vi "Picolog Thermocouple Basic.vi"() -> ()   [LabVIEW 2017]
uses:
  Controls/Thermocouple.ctl
  Controls/Temperature Units.ctl
  Controls/Fill Missing.ctl
  Controls/State Control.ctl
panel:
  in  "Tab Control":enum32{"Configuration", "Results"}(tab)=enum."Results"
  in  "Thermocouples":T1[](array[typedef])=[107, 32, 32, 32, 32, 32, 32, 32, 32, 32] items=["B"=98, "E"=101, "J"=106, "K"=107, "N"=110, "R"=114, "S"=115, "T"=116, "Voltage"=120, "Internal"=0, "Off"=32]
  in  "Mains Frequency":i16(ring) items=["50 Hz", "60 Hz"]
  in  "Unit":T2
  in  "Sampling Interval [s]":dbl=0.20000000000000004 min=0.1 max=100.0 step=0.1 format="%#_13g"
  in  "Fill Missing Points":T3 items=["QNaN", "Previous"]
  in  "Buffer Length":i32=128
  in  "Update Rate [s]":dbl=0.20000000000000004 min=0.1 max=10.0 step=0.1
  out "Actual Interval [s]":dbl=0.20000000000000004
  out "Error":errorcluster
  out "Temperature":waveform(dbl)[](graph)=[{"t0"=timestamp(3630055576.922543 s since 1904-01-01), "dt"=0.20000000000000284, "Y"=[23.393163681030273], "attributes"=variant("NI_ChannelName"=variant(string "Cold Junction"))}, {"t0"=timestamp(3630055576.922543 s since 1904-01-01), "dt"=0.20000000000000284, "Y"=[23.27175521850586], "attributes"=variant("NI_ChannelName"=variant(string "Channel 1"))}]
  in  "Stop":bool
  # "Temperature Measurement - PicoLog Thermocouple"
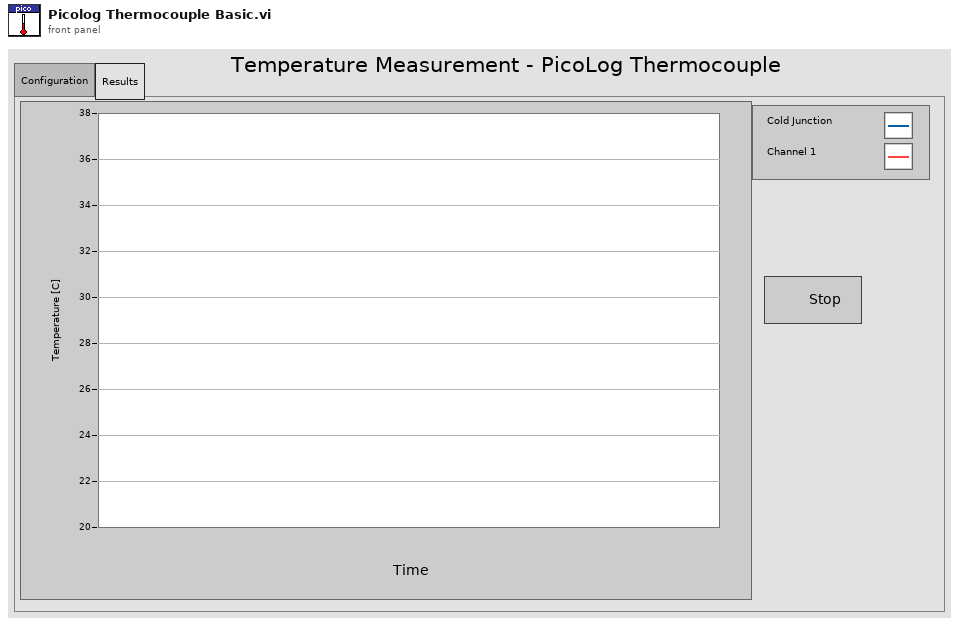
[diagram p1: front panel]
types:
  T1 = typedef "Thermocouple.ctl" = i8
  T2 = typedef "Temperature Units.ctl" = enum16{"°C", "°F", "K", "°R"}
  T3 = typedef "Fill Missing.ctl" = i16
  T4 = typedef "State Control.ctl" = enum16{"Initialize", "Idle", "Acquire", "Display", "Shutdown", "Quit", "Error"}
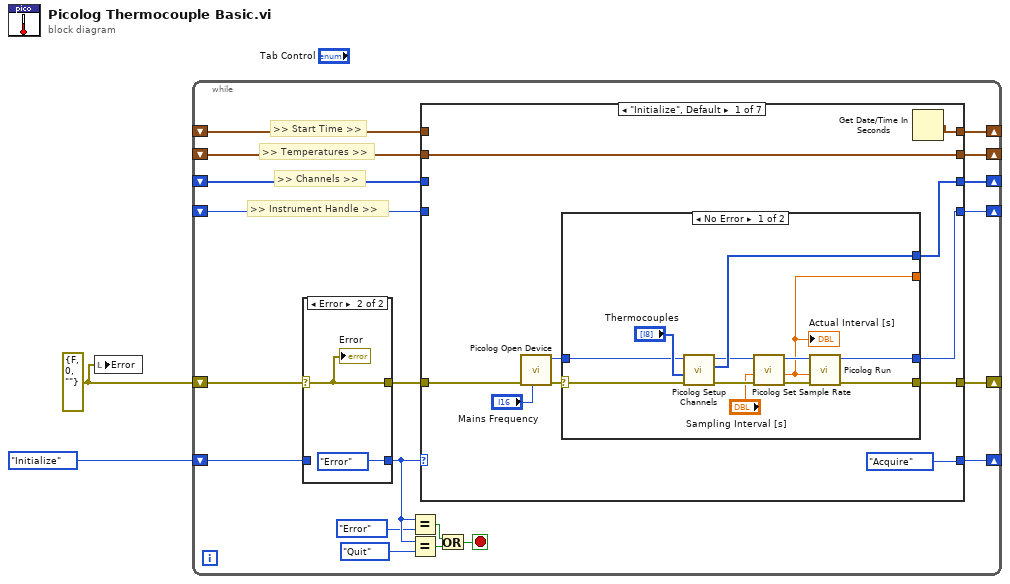
[diagram p0: block diagram]
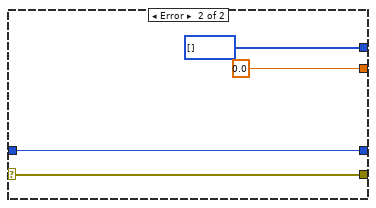
[diagram p3: hidden frame]
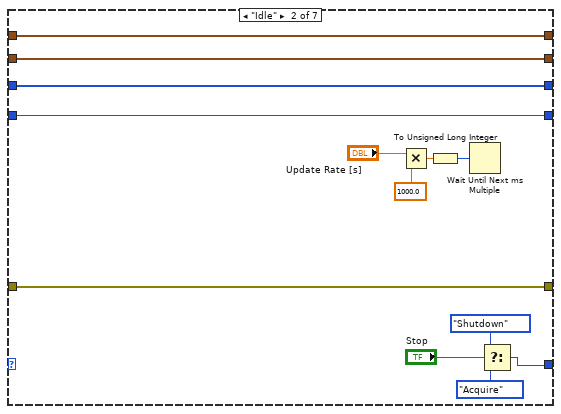
[diagram p4: hidden frame]
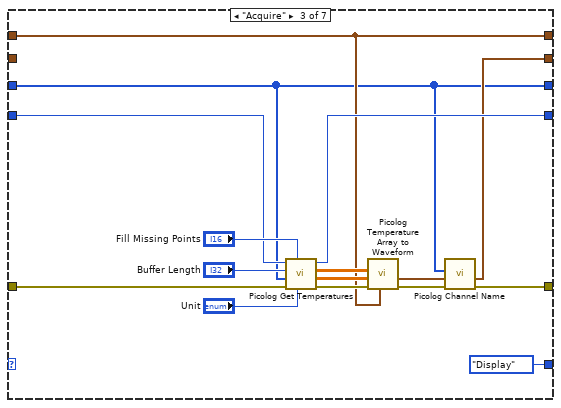
[diagram p5: hidden frame]
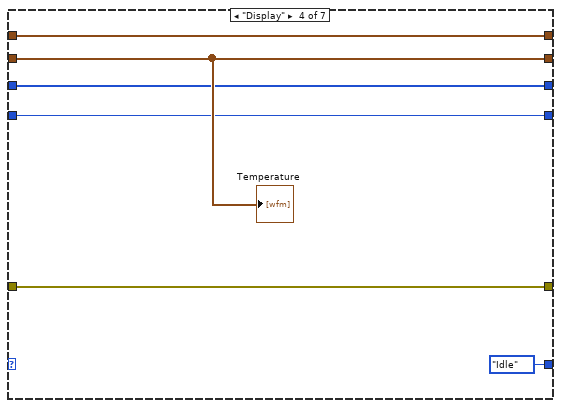
[diagram p6: hidden frame]
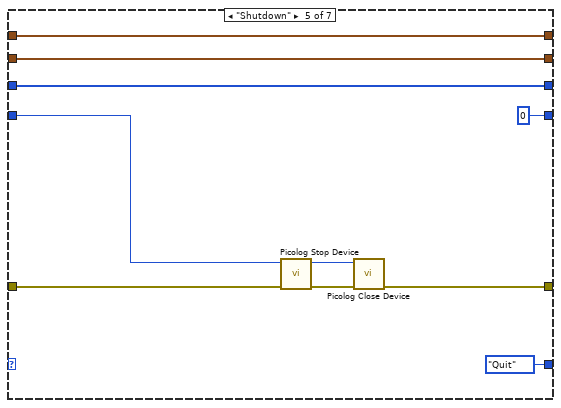
[diagram p7: hidden frame]
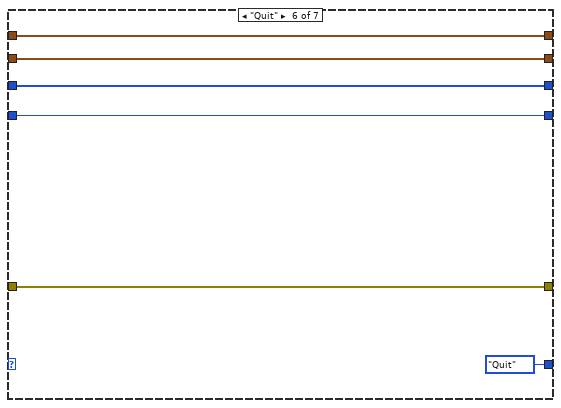
[diagram p8: hidden frame]
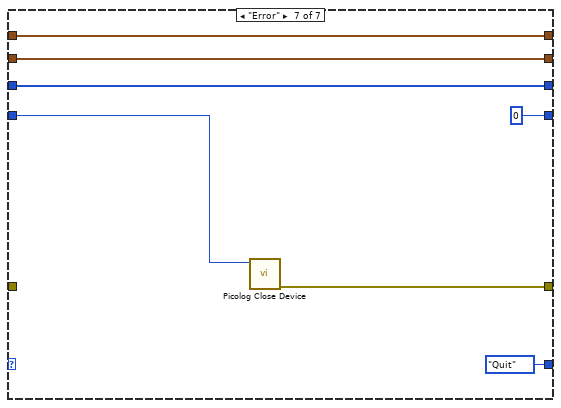
[diagram p9: hidden frame]
diagram:
  w1 = errorcluster {"status"=FALSE, "code"=0, "source"=""} ("Error Out")
  n1 = local write "Error"(w1) -> ()
  n2 = while {
    shift-right: [w12] -> _
    shift-left: _ -> [w20]
    shift-right: [w21] -> _
    shift-left: w1 -> [w5]
    shift-right: [w19] -> _
    shift-left: State_Control."Initialize" ("State") -> [w13]
    shift-right: [w18] -> _
    shift-left: _ -> [w17]
    shift-right: [w16] -> _
    shift-left: _ -> [w15]
    shift-right: [w4] -> _
    shift-left: _ -> [w3]
    stop <- w6 stop-if-true
    # ">> Start Time >>"
    # ">> Temperatures >>"
    # ">> Instrument Handle >>"
    # ">> Channels >>"
    n3 = case shown="Error" w5 {
      selector: w5 -> [w23 w24]
      tunnel: [w23 w24] -> w14
      tunnel: w13 -> [w22 _]
      tunnel: [w22 State_Control."Error" ("State")] -> w10
      frame No Error {
      }
      frame Error {
        "Error" <- w24
      }
    }
    n4 = Equal?(x=w10, y=State_Control."Error") -> (x = y?=w8:bool)
    n5 = Equal?(x=w10, y=State_Control."Quit") -> (x = y?=w7:bool)
    n6 = case shown="\"Initialize\", Default" w10 {
      tunnel: [w33 w64 w69 w84 i16 0 ("Instrument Handle Out") w98 i16 0 ("Instrument Handle Out")] -> w12
      tunnel: [w32 w63 w70 w83 w89 w99 w108] -> w21
      tunnel: w20 -> [_ w64 w71 w84 w95 w98 w109]
      tunnel: w14 -> [w31 w63 w72 w83 w96 w99 _]
      tunnel: [State_Control."Acquire" ("State") w61 State_Control."Display" ("State") State_Control."Idle" ("State") State_Control."Quit" ("State") State_Control."Quit" ("State") State_Control."Quit" ("State")] -> w19
      tunnel: [w29 w58 w68 w86 w94 w102 w105] -> w18
      tunnel: w17 -> [_ w58 w68 w86 w94 w102 w105]
      tunnel: [w28 w54 w66 w85 w92 w100 w106] -> w16
      tunnel: w15 -> [w28 w54 _ w85 w92 w100 w106]
      tunnel: [w26 w53 w65 w81 w87 w97 w103] -> w4
      tunnel: w3 -> [_ w53 w65 w81 w87 w97 w103]
      frame "Initialize", Default {
        n7 = call "Picolog Open Device.vi"("Mains Frequency"="Mains Frequency", "Error In"=w31) -> ("Error Out"=w27:errorcluster, "Instrument Handle Out"=w34:i16)  [unwired: 8 in]
        n8 = case shown="No Error" w27 {
          selector: w27 -> [w40 w51]
          tunnel: w34 -> [w43 w50]
          tunnel: [w42 w50] -> w33
          tunnel: [w41 w51] -> w32
          tunnel: [w36 0.0] -> _
          tunnel: [w39 i16[] [] ("Channels")] -> w26
          frame No Error {
            n9 = call "Picolog Setup Channels.vi"("Error In"=w40, "Configurations"="Thermocouples", "Instrument Handle"=w43) -> ("Error Out"=w45:errorcluster, "Channels"=w39:i16[], "Instrument Handle Out"=w38:i16)  [unwired: 6 in]
            n10 = call "Picolog Set Sample Rate.vi"("error in (no error)"=w45, "Sampling Interval [s]"="Sampling Interval [s]", "Instrument Handle In"=w38) -> ("error out"=w47:errorcluster, "Actual Sampling Interval [s]"=w36:dbl, "Instrument Handle Out"=w46:i16)  [unwired: 6 in]
            "Actual Interval [s]" <- w36
            n11 = call "Picolog Run.vi"("Error In"=w47, "Interval [s]"=w36, "Instrument Handle In"=w46) -> ("Error Out"=w41:errorcluster, "Instrument Handle Out"=w42:i16)  [unwired: 6 in, 1 out]
          }
          frame Error {
          }
        }
        n12 = Get Date/Time In Seconds() -> (seconds since 1Jan1904=w29:timestamp)
      }
      frame "Idle" {
        n13 = Multiply(x="Update Rate [s]", y=1000.0) -> (x*y=w56:dbl)
        n14 = To Unsigned Long Integer(number=w56) -> (unsigned 32bit integer=w55:u32)
        n15 = Wait Until Next ms Multiple(millisecond multiple=w55) -> ()  [unwired: 1 out]
        n16 = Select(t=State_Control."Shutdown" ("State"), s="Stop", f=State_Control."Acquire" ("State")) -> (s? t:f=w61:T4)
      }
      frame "Acquire" {
        n17 = call "Picolog Get Temperatures.vi"("Units"="Unit", "Fill Missing Points"="Fill Missing Points", "Error In"=w72, "Channels"=w65, "Buffer Length"="Buffer Length", "Instrument Handle In"=w71) -> ("Error Out"=w77:errorcluster, "Temperature"=w78:sgl[][], "Time [s]"=w79:dbl[][], "Instrument Handle Out"=w69:i16)  [unwired: 1 in, 1 out]
        n18 = call "Picolog Temperature Array to Waveform.vi"("Start Time"=w68, "Error In"=w77, "Temperatures"=w78, "Times [s]"=w79) -> ("Error Out"=w75:errorcluster, "Temperature Waveforms"=w76:waveform(dbl)[])  [unwired: 6 in]
        n19 = call "Picolog Channel Name.vi"("Error In"=w75, "Temperature Waveforms"=w76, "Channels"=w65) -> ("Error Out"=w70:errorcluster, "Temperature Waveforms with Names"=w66:waveform(dbl)[])  [unwired: 7 in]
      }
      frame "Display" {
        "Temperature" <- w85
      }
      frame "Shutdown" {
        n20 = call "Picolog Stop Device.vi"("Error In"=w96, "Instrument Handle In"=w95) -> ("Error Out"=w90:errorcluster, "Instrument Handle Out"=w91:i16)  [unwired: 8 in]
        n21 = call "Picolog Close Device.vi"("Error In"=w90, "Instrument Handle"=w91) -> ("Error Out"=w89:errorcluster)  [unwired: 9 in]
      }
      frame "Quit" {
      }
      frame "Error" {
        n22 = call "Picolog Close Device.vi"("Instrument Handle"=w109) -> ("Error Out"=w108:errorcluster)  [unwired: 10 in]
      }
    }
    n23 = Or(x=w8, y=w7) -> (x .or. y?=w6:bool)
  }
